vi "manageStatistics.vi"(8 "errorIn":errorcluster, 11 "state [init]":string="init") -> (0 "errorOut":errorcluster, 3 "statistics":cluster{cluster{"X":dbl, "Y":dbl}[]}[](array[cluster]))   [LabVIEW 2025]
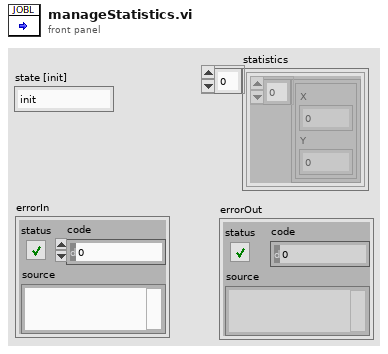
[diagram p1: front panel]
types:
  T1 = typedef "statisticsData.ctl" = cluster{"date":dbl[], "data":cluster{"index":i32, "title":string, "link":string, "salary":string, "employer":string, "employerLink":string, "level":string, "workplace":string, "keywords":string, "userNote":string, "userNote2":string, "userNote3":string, "userNote4":string, "userNote5":string}[][]}
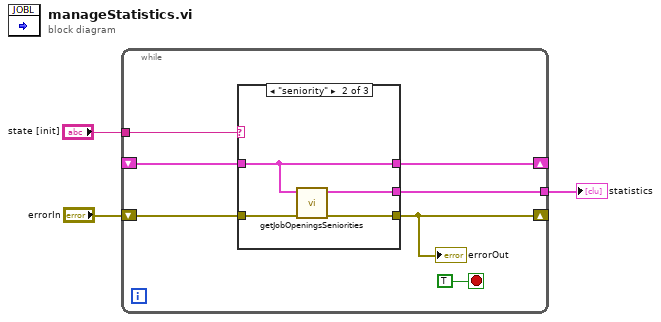
[diagram p0: block diagram]
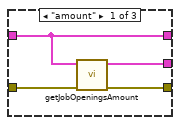
[diagram p2: hidden frame]
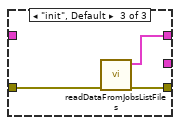
[diagram p3: hidden frame]
diagram:
  n1 = while {
    shift-right: [w9] -> _
    shift-left: _ -> [w8]
    shift-right: [w7] -> _
    shift-left: "errorIn" -> [w6]
    tunnel: "state [init]" -> [w10]
    tunnel: [w4] -> w1
    stop <- TRUE stop-if-true
    n2 = case shown="\"seniority\"" w10 {
      tunnel: [w14 w16 w21] -> w9
      tunnel: w8 -> [w14 w16 _]
      tunnel: [w11 w17 w20] -> w7
      tunnel: w6 -> [w12 w18 w19]
      tunnel: [w13 w15 _] -> w4
      frame "amount" {
        n3 = call "getJobOpeningsAmount.vi"("errorIn"=w12, "staisticsData"=w14) -> ("errorOut"=w11:errorcluster, "statistics"=w13:cluster{cluster{"X":dbl, "Y":dbl}[]}[])  [unwired: 8 in]
      }
      frame "seniority" {
        n4 = call "getJobOpeningsSeniorities.vi"("errorIn"=w18, "staisticsData"=w16) -> ("errorOut"=w17:errorcluster, "statistics"=w15:cluster{cluster{"X":dbl, "Y":dbl}[]}[])  [unwired: 8 in]
      }
      frame "init", Default {
        n5 = call "readDataFromJobsListFiles.vi"("errorIn"=w19) -> ("errorOut"=w20:errorcluster, "staitisticsData"=w21:T1)  [unwired: 9 in]
      }
    }
    "errorOut" <- w7
  }
  "statistics" <- w1
